vi "XY Graph Are Tool Panels Visible.vi"(8 "Error In":errorcluster, 11 "XY Graph Ref":T1) -> (0 "Error Out":errorcluster, 1 "Any Panel Visible?":bool, 2 "Graph Tool Panels Visibility":T2, 3 "XY Graph Ref dup":T1)   [LabVIEW 2021, in "XY Graph Add-Ons.lvlib"]
uses:
  XY Graph Add-Ons.lvlib
  XY Graph Refnum.ctl
  XY Graph Tool Panels Visibility.ctl
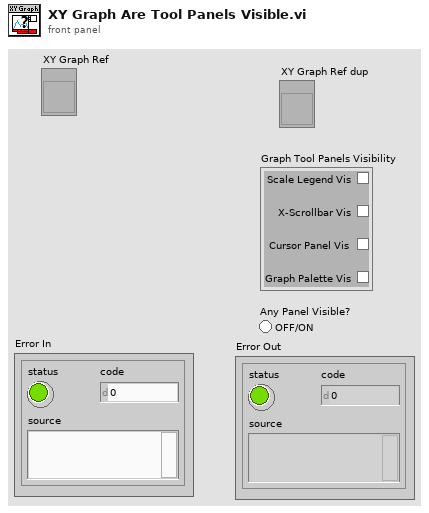
[diagram p1: front panel]
types:
  T1 = typedef "XY Graph Add-Ons.lvlib/XY Graph Refnum.ctl" = refnum<vi>
  T2 = typedef "XY Graph Add-Ons.lvlib/XY Graph Tool Panels Visibility.ctl" = cluster{"Scale Legend Vis":bool, "X-Scrollbar Vis":bool, "Cursor Panel Vis":bool, "Graph Palette Vis":bool}
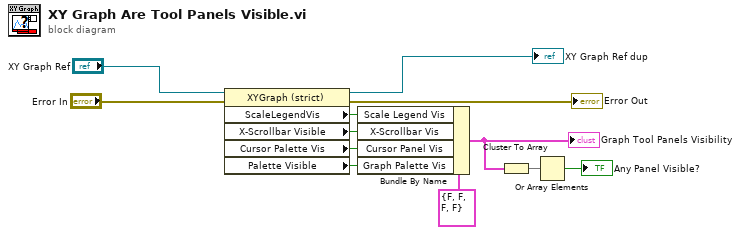
[diagram p0: block diagram]
diagram:
  n1 = property class="XYGraph (strict)"(reference="XY Graph Ref", error in="Error In") -> (reference out=→"XY Graph Ref dup":T1, error out=→"Error Out":errorcluster, "ScaleLegendVis"=w9:bool, "X-Scrollbar Visible"=w8:bool, "Cursor Palette Vis"=w7:bool, "Palette Visible"=w6:bool)
  n2 = Bundle By Name(cluster=T2 {"Scale Legend Vis"=FALSE, "X-Scrollbar Vis"=FALSE, "Cursor Panel Vis"=FALSE, "Graph Palette Vis"=FALSE} ("Graph Tool Panels Visibility"), "Scale Legend Vis"=w9, "X-Scrollbar Vis"=w8, "Cursor Panel Vis"=w7, "Graph Palette Vis"=w6) -> (w4:T2)
  "Graph Tool Panels Visibility" <- w4
  n3 = Cluster To Array(cluster=w4) -> (array=w3:bool[])
  n4 = Or Array Elements(Boolean array=w3) -> (logical OR=→"Any Panel Visible?":bool)
